vi "Upload File from Stream.vi"(4 "attributes":refnum<class "File Attributes.lvclass">, 6 "timeout (ms)":i32=30000, 8 "error in":errorcluster, 9 "remote path":string, 10 "channel":T1, 11 "session in":refnum<class "Session.lvclass">) -> (0 "error out":errorcluster, 3 "session out":refnum<class "Session.lvclass">)   [LabVIEW 2020, in "NI_SFTP.lvlib"]
doc: "Creates a new remote file, initialized with a High-Speed Stream of byte arrays."
uses:
  <vilib>/net/SFTP/NI_SFTP.lvlib
  <vilib>/net/SFTP/File Attributes/File Attributes.lvclass
  <vilib>/net/SFTP/Session/Session.lvclass
  <extravilib>/ChannelInstances/High Speed Stream-a[.](u8)/)Channel.ctl
  <extravilib>/ChannelInstances/High Speed Stream-a[.](u8)/_Read For Replicate.vi
  <extravilib>/ChannelInstances/High Speed Stream-a[.](u8)/)Channel.vi
  <extravilib>/ChannelInstances/High Speed Stream-a[.](u8)/Abort Signal/Init Signal.vi
  <vilib>/net/SFTP/API/Support/Upload/Stream/Stream Upload Controller.lvclass
  <extravilib>/ChannelInstances/High Speed Stream-a[.](u8).lvlib
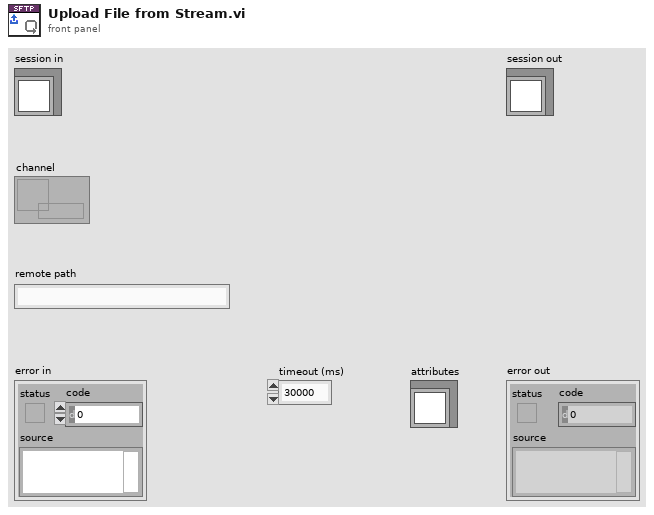
[diagram p1: front panel]
types:
  T1 = typedef "High Speed Stream-a[.](u8).lvlib/)Channel.ctl" = refnum<queue>
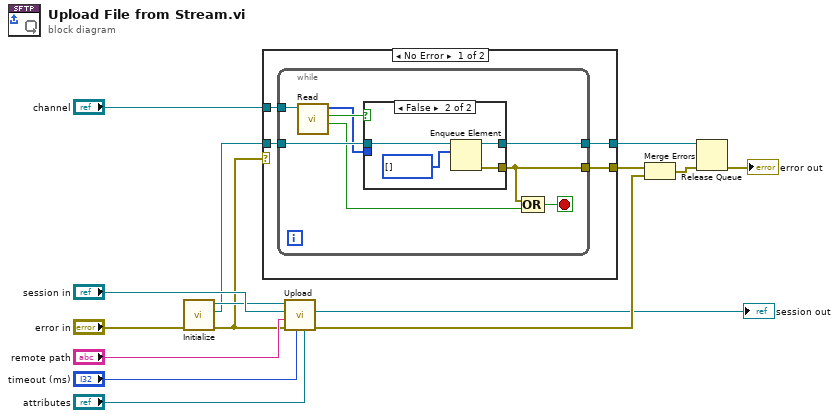
[diagram p0: block diagram]
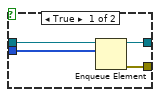
[diagram p2: hidden frame]
diagram:
  n1 = call <vilib>:"Initialize.vi"("error in (no error)"="error in") -> ("error out"=w7:errorcluster, "queue out"=w9:refnum<queue>, "Stream Upload Controller out"=w10:refnum<class "Stream Upload Controller.lvclass">)  [unwired: 8 in]
  n2 = case shown="No Error" w7 {
    tunnel: w9 -> [w19 w36]
    tunnel: "channel" -> [w18 _]
    tunnel: [w17 w36] -> w4
    tunnel: [w16 _] -> w6
    frame No Error {
      n3 = while {
        tunnel: w19 -> [w26]
        tunnel: w18 -> [w27]
        tunnel: [w24] -> w17
        tunnel: [w21] -> w16
        stop <- w22 stop-if-true
        n4 = call <extravilib>:"Read.vi"("channel"=w27) -> ("done?"=w23:bool, "element valid?"=w25:bool, "element"=w20:u8[])  [unwired: 6 in, 2 out]
        n5 = case shown="False" w25 {
          tunnel: w26 -> [w31 w35]
          tunnel: [w30 w34] -> w24
          tunnel: [w29 w33] -> w21
          tunnel: w20 -> [w28 _]
          frame True {
            n6 = Enqueue Element(queue=w31, element=w28) -> (queue out=w30:refnum<queue>, error out=w29:errorcluster)  [unwired: 2 in, 1 out]
          }
          frame False {
            n7 = Enqueue Element(queue=w35, element=u8[] []) -> (queue out=w34:refnum<queue>, error out=w33:errorcluster)  [unwired: 2 in, 1 out]
          }
        }
        n8 = Compound Arithmetic op=OR(w21, w23) -> (w22:bool)
      }
    }
    frame Error {
    }
  }
  n9 = call-dynamic "Upload.vi"("attributes"="attributes", "timeout (ms)"="timeout (ms)", "error in"=w7, "remote path"="remote path", "session in"="session in", "NI_SFTP.lvlib:Generic Upload Controller.lvclass"=w10) -> ("error out"=w5:errorcluster, "session out"=→"session out":refnum<class "Session.lvclass">)  [unwired: 3 in, 1 out]
  n10 = Merge Errors(w6, w5) -> (w3:errorcluster)
  n11 = Release Queue(queue=w4, error in (no error)=w3) -> (error out=→"error out":errorcluster)  [unwired: 1 in, 2 out]
